vi "Log.vi"(11 "Log in":string) -> ()   [LabVIEW 2019]
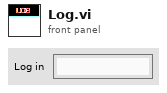
[diagram p1: front panel]
types:
  T1 = enum16{"open", "replace", "create", "open or create", "replace or create", "replace or create with confirmation"}
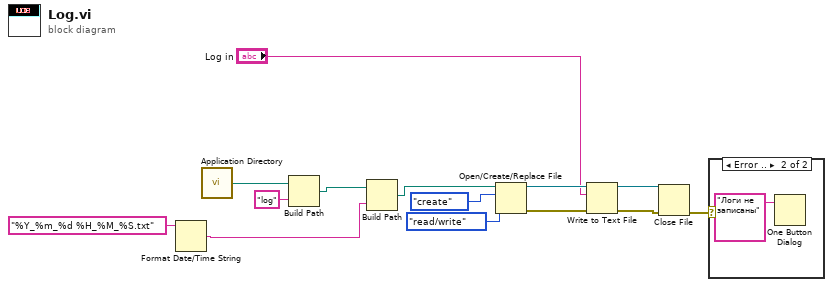
[diagram p0: block diagram]
diagram:
  n1 = Format Date/Time String(time format string (%c)="%Y_%m_%d %H_%M_%S.txt") -> (date/time string=w2:string)  [unwired: 2 in]
  n2 = call <vilib>:"Application Directory.vi"() -> ("Application Directory"=w14:path)
  n3 = Build Path(base path=w14, name or relative path="log") -> (appended path=w12:path)
  n4 = Build Path(base path=w12, name or relative path=w2) -> (appended path=w8:path)
  n5 = Open/Create/Replace File(file path (use dialog)=w8, operation (0:open)=T1."create", access (0:read/write)=enum16{"read/write", "read-only", "write-only"}."read/write") -> (refnum out=w11:refnum<file>, error out=w10:errorcluster)  [unwired: 3 in, 1 out]
  n6 = Write to Text File(file (use dialog)=w11, text="Log in", error in=w10) -> (refnum out=w6:refnum<file>, error out=w5:errorcluster)  [unwired: 1 in, 1 out]
  n7 = Close File(refnum=w6, error in=w5) -> (error out=w1:errorcluster)  [unwired: 1 out]
  n8 = case shown="Error .." w1 {
    frame No Error {
    }
    frame Error {
      n9 = One Button Dialog(message="Логи не записаны") -> ()  [unwired: 1 in, 1 out]
    }
  }
